vi "Set Splitter Style (Core).vi"(8 "error in (no error)":errorcluster, 10 "Style":T1 items=["Modern", "Classic", "System", "NXG"], 11 "Splitter in":refnum<class "Splitter.lvclass">) -> (0 "error out":errorcluster, 3 "Splitter out":refnum<class "Splitter.lvclass">)   [LabVIEW 2015, in "Splitter.lvclass"]
uses:
  Splitter.lvclass
  Typedefs/Splitter Style--Enum.ctl
  Splitter.lvclass/Splitter.ctl
  Low-Level VI Manipulation/Find Resource by Type (String).vi
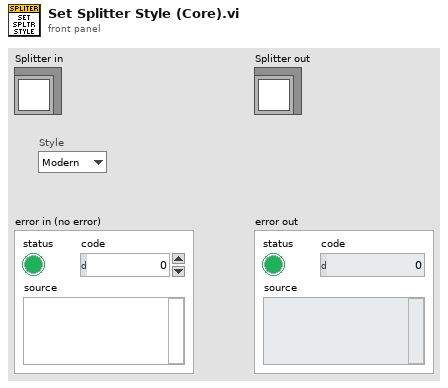
[diagram p1: front panel]
types:
  T1 = typedef "Splitter Style--Enum.ctl" = u16
  T2 = enum16{"Parse Style", "Update Style", "Store XML"}
  T3 = typedef "Resource Array.ctl" = T4[]
  T4 = typedef "Resource.ctl" = cluster{"type":u32, "id":i32, "name":string, "binary data":string}
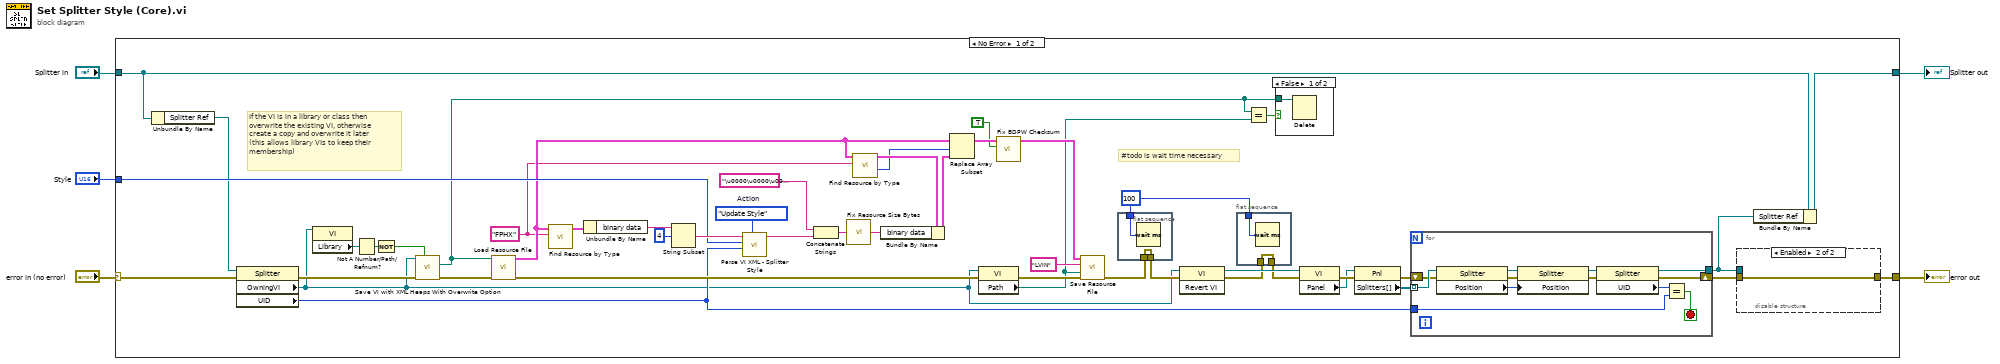
[diagram p0: block diagram]
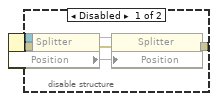
[diagram p3: hidden frame]
diagram:
  n1 = case shown="No Error" "error in (no error)" {
    selector: "error in (no error)" -> [w50 w78]
    tunnel: [w32 w78] -> w4
    tunnel: [w23 w79] -> w2
    tunnel: "Splitter in" -> [w22 w79]
    tunnel: "Style" -> [w48 _]
    frame No Error {
      w8 = T2."Update Style"  # Action
      w20 = u32 100 ("milliseconds to wait")
      w33 = "FPHX"
      # "If the VI is in a library or class then overwrite the existing VI, otherwise create a copy and overwrite it later (this allows library VIs to keep their membership)"
      # "#todo is wait time necessary"
      n2 = Unbundle By Name(w22) -> ("Splitter Ref"=w24:refnum<vi>)
      n3 = property class="Splitter"(reference=w24, error in=w50) -> (error out=w15:errorcluster, "OwningVI"=w13:refnum<vi>, "UID"=w26:i32)  [unwired: 1 out]
      n4 = property class="VI"(reference=w13) -> ("Library"=w7:refnum<vi>)  [unwired: 1 in, 2 out]
      n5 = Not A Number/Path/Refnum?(number/path/refnum=w7) -> (NaN/Path/Refnum?=w6:bool)
      n6 = Not(x=w6) -> (.not. x?=w12:bool)
      n7 = call "Save VI with XML Heaps With Overwrite Option.vi"("Overwrite VI?"=w12, "error in (no error)"=w15, "VI Refnum In"=w13) -> ("error out"=w14:errorcluster, "VI Path out"=w9:path)  [unwired: 6 in, 1 out]
      n8 = call "Load Resource File.vi"("error in (no error)"=w14, "Resource file"=w9) -> ("error out"=w38:errorcluster, "Resources"=w36:T3)  [unwired: 7 in, 1 out]
      n9 = call-poly "Find Resource by Type.vi"("Resource Type"=w33, "Resources"=w36) -> ("Resource"=w51:T4)  [unwired: 7 in, 2 out]
      n10 = Unbundle By Name(w51) -> ("binary data"=w52:string)
      n11 = String Subset(string=w52, offset (0)=4) -> (substring=w49:string)  [unwired: 1 in]
      n12 = call "Parse VI XML - Splitter Style.vi"("Action"=w8, "UID"=w26, "New Style"=w48, "VI XML in"=w49) -> ("VI XML out"=w37:string)  [unwired: 4 in, 1 out]
      n13 = Concatenate Strings("\u0000\u0000\u0000\u0000", w37) -> (w46:string)
      n14 = call "Fix Resource Size Bytes.vi"("Data In"=w46) -> ("Data Out"=w45:string)
      n15 = call-poly "Find Resource by Type.vi"("Resource Type"=w33, "Resources"=w36) -> ("Index"=w43:i32, "Resource"=w44:T4)  [unwired: 7 in, 1 out]
      n16 = Bundle By Name(cluster=w44, "binary data"=w45) -> (w42:T4)
      n17 = Replace Array Subset(array=w36, new element=w42, index=w43) -> (w41:T3)
      n18 = property class="VI"(reference=w13, error in=w38) -> (error out=w34:errorcluster, "Path"=w11:path)  [unwired: 1 out]
      n19 = call "Fix BDPW Checksum.vi"("Only fix 3rd hash (F)"=TRUE, "Resources in"=w41) -> ("Resources out"=w40:T3)  [unwired: 9 in]
      n20 = call "Save Resource File.vi"("error in (no error)"=w34, "Path"=w11, "File type"="LVIN", "Resources"=w40) -> ("error out"=w18:errorcluster)  [unwired: 7 in]
      n21 = flat-sequence {
        tunnel: w20 -> [w57]
        tunnel: [w56] -> w19
        tunnel: w18 -> [w56]
        frame #0 {
          n22 = Wait (ms)(milliseconds to wait=w57) -> ()  [unwired: 1 out]
        }
      }
      n23 = invoke class="VI" method="Revert VI"(reference=w13, error in=w19) -> (reference out=w31:refnum<vi>, error out=w16:errorcluster)  [unwired: 1 in, 1 out]
      n24 = flat-sequence {
        tunnel: w20 -> [w55]
        tunnel: [w54] -> w17
        tunnel: w16 -> [w54]
        frame #0 {
          n25 = Wait (ms)(milliseconds to wait=w55) -> ()  [unwired: 1 out]
        }
      }
      n26 = Equal?(x=w9, y=w11) -> (x = y?=w10:bool)
      n27 = case shown="False" w10 {
        tunnel: w9 -> [w58 _]
        frame False {
          n28 = Delete(path (use dialog)=w58) -> ()  [unwired: 4 in, 3 out]
        }
        frame True {
        }
      }
      n29 = property class="VI"(reference=w31, error in=w17) -> (error out=w30:errorcluster, "Panel"=w29:refnum<vi>)  [unwired: 1 out]
      n30 = property class="Pnl"(reference=w29, error in=w30) -> (error out=w28:errorcluster, "Splitters[]"=w27:refnum<vi>[])  [unwired: 1 out]
      n31 = for {
        tunnel: w27 -> [w68] mode=indexing
        tunnel: w26 -> [w76]
        shift-right: [w74] -> w25
        shift-left: w28 -> [w66]
        tunnel: [w73] -> w21
        stop <- w75 stop-if-true
        n32 = property class="Splitter"(reference=w68, error in=w66) -> (reference out=w71:refnum<vi>, error out=w72:errorcluster, "Position"=w70:i32)
        n33 = property class="Splitter"(reference=w71, error in=w72, "Position"=w70) -> (reference out=w69:refnum<vi>, error out=w67:errorcluster)
        n34 = property class="Splitter"(reference=w69, error in=w67) -> (reference out=w73:refnum<vi>, error out=w74:errorcluster, "UID"=w77:i32)
        n35 = Equal?(x=w77, y=w76) -> (x = y?=w75:bool)
      }
      n36 = disable-structure shown="Enabled" {
        disable-tunnel: [w61 w65] -> w32
        disable-tunnel: w25 -> [w60 w65]
        disable-tunnel: w21 -> [w59 _]
        frame Disabled {
          n37 = property class="Splitter"(reference=w59, error in=w60) -> (reference out=w63:refnum<vi>, error out=w62:errorcluster, "Position"=w64:i32)
          n38 = property class="Splitter"(reference=w63, error in=w62, "Position"=w64) -> (error out=w61:errorcluster)  [unwired: 1 out]
        }
        frame Enabled {
        }
      }
      n39 = Bundle By Name(cluster=w22, "Splitter Ref"=w21) -> (w23:refnum<class "Splitter.lvclass">)
    }
    frame Error {
    }
  }
  "error out" <- w4
  "Splitter out" <- w2
